vi "playback.vi"() -> ()   [LabVIEW 2012]
doc: "This VI will initialize the FPGA VI and read a user-defined number of samples from a DMA FIFO. When the data acquisition is complete this VI will read status information from the FPGA VI.\n\nFollow these instructions to run the VI.\n\n1. Select your RIO device from the dropdown.\n2. Set the sample period, number of samples to acquire per channel, and DMA block read size. \n\nNote: the block read size should be set to balance load on the host processor and the update rate of the user interface. A small block read size will update the user interface more often but will result in a higher load on the host processor."
uses:
  <vilib>/Analysis/3filter.llb/Butterworth Filter (DBL).vi
  <vilib>/Analysis/NI_AALBase.lvlib
  <vilib>/Analysis/NI_AALPro.lvlib
panel:
  in  "Wait?":bool
  in  "Filename":path=path "D:/Recorded/US Test/Record 1/Robosub.tdms"
  in  "Next Signal":bool
  in  "threshold ratio":dbl=3.0
  out "Sidemove":dbl
  out "Forward":dbl
  out "Threshold 3":dbl
  out "Threshold 2":dbl
  out "Threshold 1":dbl
  out "noise index":dbl[](array[numeric])
  out "Threshold 0":dbl
  out "Amplitude Spectrum":waveform(dbl)(graph)
  out "bad signal?":bool
  in  "Min Starting Index":i32=7000
  in  "Portion Duration":i32=1000
  out "amplitude 3":dbl
  out "amplitude 2":dbl
  out "amplitude 1":dbl
  out "amplitude 0":dbl
  in  "noise min":dbl=0.001
  out "Index 3":dbl
  out "Index 2":dbl
  out "Index 1":dbl
  out "Index 0":dbl
  in  "Send to ROS":bool
  out "ROS  Error":bool
  out "dt1":dbl
  out "dt2":dbl
  out "dt3":dbl
  out "pitch":dbl
  out "yaw":dbl
  out "z":dbl
  out "y":dbl format="%#_6f"
  out "x":dbl format="%#_6f"
  in  "Mode":T1(ring)=enum."Use Far Field"
  in  "Altitude":dbl=2.0
  in  "Display Filtered Signal":bool=TRUE
  out "Ratio at Index (%)":dbl
  out "Selected Index":i32
  in  "Threshold":dbl=0.1
  in  "low cutoff freq: fl":dbl=20000.0
  in  "high cutoff freq: fh":dbl=30000.0
  out "Yaw Chart":dbl(graph)
  out "Ch0 Signal":dbl[](graph)
  out "Extracted signal":dbl[][](graph)
  # "Peak Finding"
  # "Setpoints"
  # "TDOA (us)"
  # "Triangulation Result"
  # "Signal Processing Control"
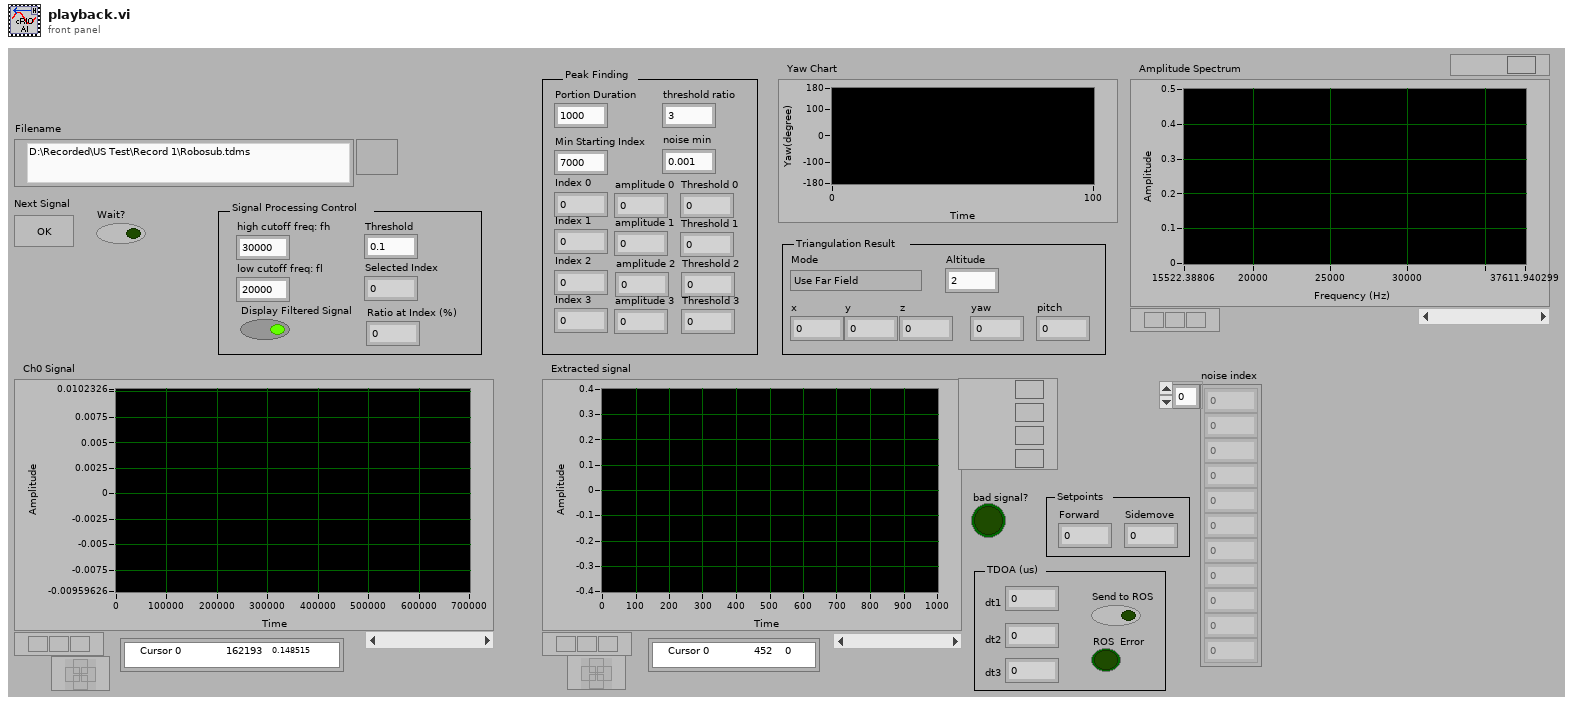
[diagram p1: front panel]
types:
  T1 = enum16{"Use Near Field", "Use Far Field", "Far Field with 3 hydrophones"}
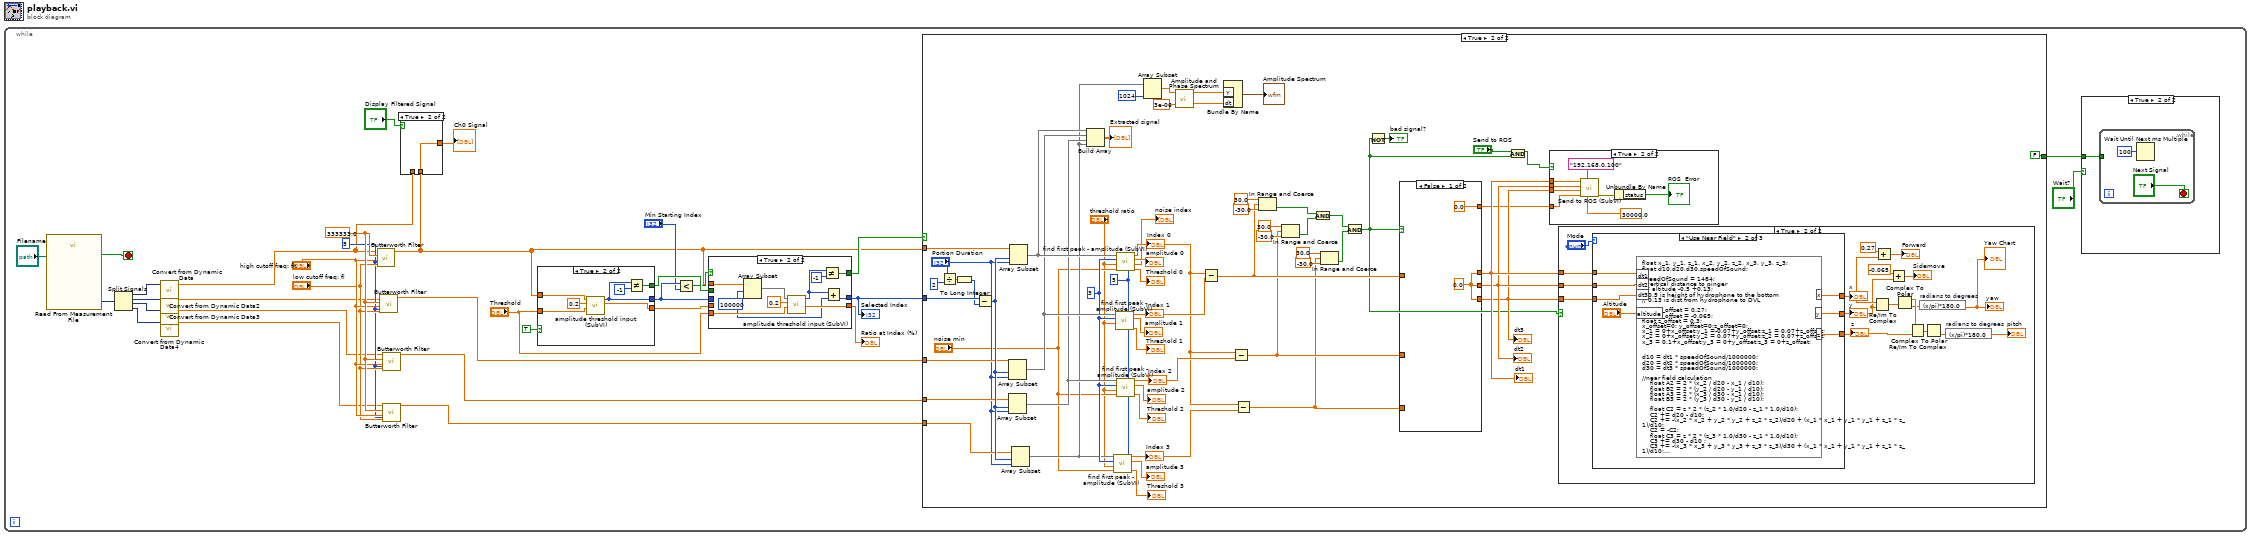
[diagram p0: block diagram]
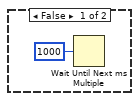
[diagram p2: hidden frame]
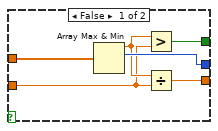
[diagram p5: hidden frame]
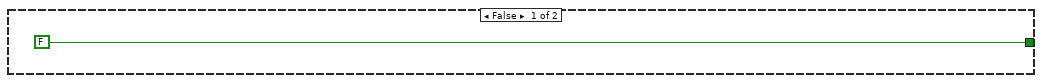
[diagram p6: hidden frame]
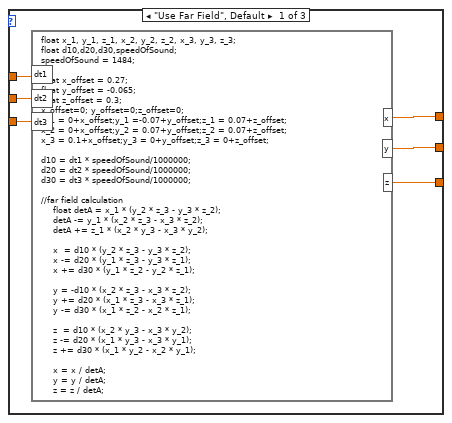
[diagram p8: hidden frame]
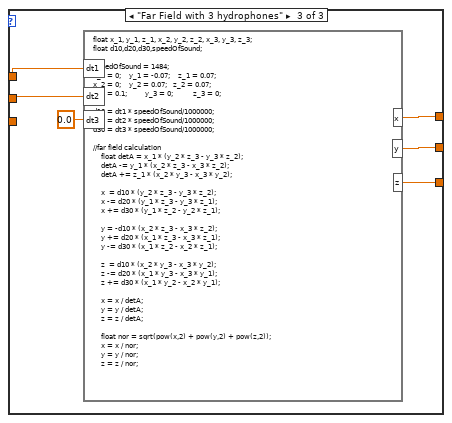
[diagram p9: hidden frame]
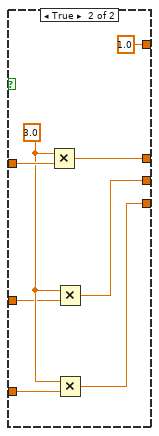
[diagram p11: hidden frame]
diagram:
  n1 = while {
    stop <- w6 stop-if-true
    w18 = 5 ("order")
    w24 = 333333.0 ("sampling freq: fs")
    n2 = call "Read From Measurement File"("Filename"="Filename") -> ("Signals"=w11:dynamicdata, "EOF?"=w6:bool)  [unwired: 5 in, 4 out]
    n3 = Split Signals(w11) -> (w15:dynamicdata, w14:dynamicdata, w13:dynamicdata, w12:dynamicdata)  [unwired: 4 in]
    n4 = call "Convert from Dynamic Data"("Dynamic Data Type"=w15) -> ("Array"=w10:dbl[])  [unwired: 3 in]
    n5 = call "Convert from Dynamic Data2"("Dynamic Data Type"=w14) -> ("Array"=w9:dbl[])  [unwired: 3 in]
    n6 = call "Convert from Dynamic Data3"("Dynamic Data Type"=w13) -> ("Array"=w7:dbl[])  [unwired: 3 in]
    n7 = call "Convert from Dynamic Data4"("Dynamic Data Type"=w12) -> ("Array"=w8:dbl[])  [unwired: 3 in]
    n8 = call-poly <vilib>:"Butterworth Filter.vi"("order"=w18, "low cutoff freq: fl"="low cutoff freq: fl", "high cutoff freq: fh"="high cutoff freq: fh", "sampling freq: fs"=w24, "X"=w10) -> ("Filtered X"=w16:dbl[])  [unwired: 3 in, 1 out]
    n9 = call-poly <vilib>:"Butterworth Filter.vi"("order"=w18, "low cutoff freq: fl"="low cutoff freq: fl", "high cutoff freq: fh"="high cutoff freq: fh", "sampling freq: fs"=w24, "X"=w9) -> ("Filtered X"=w21:dbl[])  [unwired: 3 in, 1 out]
    n10 = call-poly <vilib>:"Butterworth Filter.vi"("order"=w18, "low cutoff freq: fl"="low cutoff freq: fl", "high cutoff freq: fh"="high cutoff freq: fh", "sampling freq: fs"=w24, "X"=w8) -> ("Filtered X"=w19:dbl[])  [unwired: 3 in, 1 out]
    n11 = call-poly <vilib>:"Butterworth Filter.vi"("order"=w18, "low cutoff freq: fl"="low cutoff freq: fl", "high cutoff freq: fh"="high cutoff freq: fh", "sampling freq: fs"=w24, "X"=w7) -> ("Filtered X"=w20:dbl[])  [unwired: 3 in, 1 out]
    n12 = case shown="True" "Display Filtered Signal" {
      tunnel: w10 -> [w38 _]
      tunnel: [w38 w39] -> w4
      tunnel: w16 -> [_ w39]
      frame False {
      }
      frame True {
      }
    }
    "Ch0 Signal" <- w4
    n13 = case shown="True" TRUE {
      tunnel: w16 -> [w58 w65]
      tunnel: [w55 w62] -> w30
      tunnel: [w56 w61] -> w27
      tunnel: [w57 w60] -> w32
      tunnel: "Threshold" -> [w53 w59]
      frame False {
        n14 = Array Max & Min(array=w58) -> (max value=w54:dbl, max index (indices)=w56:i32)  [unwired: 2 out]
        n15 = Greater?(x=w54, y=w53) -> (0:w57:bool)
        n16 = Divide(x=w54, y=w53) -> (x/y=w55:dbl)
      }
      frame True {
        n17 = call "amplitude threshold input (SubVI).vi"("threshold"=w59, "%max amplitude"=0.2, "Array"=w65) -> ("actual ratio (%)"=w62:dbl, "Index"=w61:i32)  [unwired: 7 in]
        n18 = Not Equal?(x=w61, y=-1) -> (x != y?=w60:bool)
      }
    }
    n19 = Less?(x=w27, y="Min Starting Index") -> (x < y?=w31:bool)
    n20 = case shown="True" w31 {
      tunnel: w32 -> [w42 _]
      tunnel: w30 -> [w40 _]
      tunnel: w16 -> [_ w52]
      tunnel: "Threshold" -> [_ w48]
      tunnel: [w42 w47] -> w25
      tunnel: [w41 w45] -> w26
      tunnel: [w40 w46] -> w28
      tunnel: w27 -> [w41 _]
      frame False {
      }
      frame True {
        w43 = 100000 ("index")
        n21 = Array Subset(array=w52, index=w43) -> (w49:dbl[])  [unwired: 1 in]
        n22 = call "amplitude threshold input (SubVI).vi"("threshold"=w48, "%max amplitude"=0.2, "Array"=w49) -> ("actual ratio (%)"=w46:dbl, "Index"=w44:i32)  [unwired: 7 in]
        n23 = Not Equal?(x=w44, y=-1) -> (x != y?=w47:bool)
        n24 = Add(x=w44, y=w43) -> (x+y=w45:i32)
      }
    }
    "Ratio at Index (%)" <- w28
    "Selected Index" <- w26
    n25 = case shown="True" w25 {
      tunnel: w21 -> [_ w125]
      tunnel: w20 -> [_ w124]
      tunnel: w19 -> [_ w123]
      tunnel: w16 -> [_ w122]
      tunnel: w26 -> [_ w121]
      tunnel: [FALSE ("Debug") FALSE ("Debug")] -> w3
      frame False {
      }
      frame True {
        w74 = 5 ("Noise length")
        w87 = 3
        n26 = Divide(x="Portion Duration", y=2) -> (x/y=w118:dbl)
        n27 = To Long Integer(number=w118) -> (32bit integer=w117:i32)
        n28 = Subtract(x=w121, y=w117) -> (x-y=w126:i32)
        n29 = Array Subset(array=w124, index=w126, length="Portion Duration") -> (w88:dbl[])
        n30 = Array Subset(array=w125, index=w126, length="Portion Duration") -> (w92:dbl[])
        n31 = Array Subset(array=w122, index=w126, length="Portion Duration") -> (w94:dbl[])
        n32 = Array Subset(array=w123, index=w126, length="Portion Duration") -> (w86:dbl[])
        n33 = Build Array(w94, w92, w88, w86) -> (→"Extracted signal":dbl[][])
        n34 = call "find first peak - amplitude (SubVI).vi"("Noise length"=w74, "Noise min"="noise min", "threshold ratio"="threshold ratio", "width"=w87, "Array"=w86) -> ("Peak threshold"=→"Threshold 3":dbl, "peak amplitude"=→"amplitude 3":dbl, "Index"=w85:dbl)  [unwired: 2 in, 2 out]
        "Index 3" <- w85
        n35 = call "find first peak - amplitude (SubVI).vi"("Noise length"=w74, "threshold ratio"="threshold ratio", "width"=w87, "Array"=w92) -> ("Peak threshold"=→"Threshold 1":dbl, "peak amplitude"=→"amplitude 1":dbl, "Index"=w91:dbl)  [unwired: 3 in, 2 out]
        "Index 1" <- w91
        n36 = call "find first peak - amplitude (SubVI).vi"("Noise length"=w74, "Noise min"="noise min", "threshold ratio"="threshold ratio", "width"=w87, "Array"=w94) -> ("Peak threshold"=→"Threshold 0":dbl, "noise index"=→"noise index":dbl[], "peak amplitude"=→"amplitude 0":dbl, "Index"=w81:dbl)  [unwired: 2 in, 1 out]
        "Index 0" <- w81
        n37 = call "find first peak - amplitude (SubVI).vi"("Noise length"=w74, "Noise min"="noise min", "threshold ratio"="threshold ratio", "width"=w87, "Array"=w88) -> ("Peak threshold"=→"Threshold 2":dbl, "peak amplitude"=→"amplitude 2":dbl, "Index"=w89:dbl)  [unwired: 2 in, 2 out]
        "Index 2" <- w89
        n38 = Array Subset(array=w86, length=1024) -> (w70:dbl[])  [unwired: 1 in]
        n39 = call <vilib>:"Amplitude and Phase Spectrum.vi"("dt"=3e-06, "Signal (V)"=w70) -> ("df"=w67:dbl, "Amp Spectrum Mag (Vrms)"=w68:dbl[])  [unwired: 1 in, 1 out]
        n40 = Subtract(x=w81, y=w91) -> (x-y=w113:dbl)
        n41 = Bundle By Name("Y"=w68, "dt"=w67) -> (→"Amplitude Spectrum":waveform(dbl))  [unwired: 1 in]
        n42 = Subtract(x=w81, y=w89) -> (x-y=w110:dbl)
        n43 = Subtract(x=w81, y=w85) -> (x-y=w107:dbl)
        n44 = In Range and Coerce(upper limit=30.0, x=w113, lower limit=-30.0) -> (In Range?=w106:bool)  [unwired: 1 out]
        n45 = In Range and Coerce(upper limit=30.0, x=w110, lower limit=-30.0) -> (In Range?=w105:bool)  [unwired: 1 out]
        n46 = And(x=w106, y=w105) -> (x .and. y?=w104:bool)
        n47 = In Range and Coerce(upper limit=30.0, x=w107, lower limit=-30.0) -> (In Range?=w103:bool)  [unwired: 1 out]
        n48 = And(x=w104, y=w103) -> (x .and. y?=w95:bool)
        n49 = Not(x=w95) -> (.not. x?=→"bad signal?":bool)
        n50 = case shown="False" w95 {
          tunnel: w113 -> [_ w181]
          tunnel: w110 -> [_ w179]
          tunnel: w107 -> [_ w178]
          tunnel: [w172 w177] -> w100
          tunnel: [w172 w176] -> w99
          tunnel: [w172 w175] -> w98
          tunnel: [0.0 ("x") 1.0 ("x")] -> w97
          frame False {
            w172 = 0.0
          }
          frame True {
            w180 = 3.0 ("x")
            n51 = Multiply(x=w180, y=w181) -> (x*y=w177:dbl)
            n52 = Multiply(x=w180, y=w179) -> (x*y=w176:dbl)
            n53 = Multiply(x=w180, y=w178) -> (x*y=w175:dbl)
          }
        }
        "dt1" <- w100
        "dt2" <- w99
        "dt3" <- w98
        n54 = And(x="Send to ROS", y=w95) -> (x .and. y?=w96:bool)
        n55 = case shown="True" w96 {
          tunnel: w100 -> [_ w167]
          tunnel: w99 -> [_ w166]
          tunnel: w98 -> [_ w165]
          tunnel: w97 -> [_ w164]
          frame False {
          }
          frame True {
            n56 = call "Send to ROS (SubVI).vi"("frequency"=30000.0, "ROS IP"="192.168.0.100", "Good signal?"=w164, "dt 3"=w165, "dt2"=w166, "dt 1"=w167) -> ("error out"=w170:errorcluster)  [unwired: 5 in]
            n57 = Unbundle By Name(w170) -> ("status"=→"ROS  Error":bool)
          }
        }
        n58 = case shown="True" w95 {
          tunnel: w100 -> [_ w135]
          tunnel: w99 -> [_ w134]
          tunnel: w98 -> [_ w133]
          frame False {
          }
          frame True {
            n59 = case shown="\"Use Near Field\"" "Mode" {
              tunnel: [w150 w157 w162] -> w132
              tunnel: [w149 w156 w161] -> w129
              tunnel: [w148 w155 w160] -> w139
              tunnel: w135 -> [w147 w153 w159]
              tunnel: w134 -> [w146 w152 w158]
              tunnel: w133 -> [w145 w151 _]
              frame "Use Far Field", Default {
                n60 = formula code="float x_1, y_1, z_1, x_2, y_2, z_2, x_3, y_3, z_3;\nfloat d10,d20,d30,speedOfSound;\nspeedOfSound = 1484;\n\nfloat x_offset = 0.27;\nfloat y_offset = -0.065;\nfloat z_offset = 0.3;\nx_offset=0; y_offset=0;z_offset=0;\nx_1 = 0+x_offset;y_1 =-0.07+y_offset;z_1 = 0.07+z_offset;\nx_2 = 0+x_offset;y_2 = 0.07+y_offset;z_2 = 0.07+z_offset;\nx_3 = 0.1+x_offset;y_3 = 0+y_offset;z_3 = 0+z_offset;\n\nd10 = dt1 * speedOfSound/1000000;\nd20 = dt2 * speedOfSound/1000000;\nd30 = dt3 * speedOfSound/1000000;\n\n//far field calculation\n    float detA = x_1 * (y_2 * z_3 - y_3 * z_2);\n    detA -= y_1 * (x_2 * z_3 - x_3 * z_2);\n    detA += z_1 * (x_2 * y_3 - x_3 * y_2);\n\n    x  = d10 * (y_2 * z_3 - y_3 * z_2);\n    x -= d20 * (y_1 * z_3 - y_3 * z_1);\n    x += d30 * (y_1 * z_2 - y_2 * z_1);\n\n    y = -d10 * (x_2 * z_3 - x_3 * z_2);\n    y += d20 * (x_1 * z_3 - x_3 * z_1);\n    y -= d30 * (x_1 * z_2 - x_2 * z_1);\n\n    z  = d10 * (x_2 * y_3 - x_3 * y_2);\n    z -= d20 * (x_1 * y_3 - x_3 * y_1);\n    z += d30 * (x_1 * y_2 - x_2 * y_1);\n\n    x = x / detA;\n    y = y / detA;\n    z = z / detA;\n\n    float nor = sqrt(pow(x,2) + pow(y,2) + pow(z,2));\n    x = x / nor;\n    y = y / nor;\n    z = z / nor;"("dt1"=w147, "dt2"=w146, "dt3"=w145) -> ("x"=w150:dbl, "y"=w149:dbl, "z"=w148:dbl)
              }
              frame "Use Near Field" {
                n61 = formula code="float x_1, y_1, z_1, x_2, y_2, z_2, x_3, y_3, z_3;\nfloat d10,d20,d30,speedOfSound;\n\nspeedOfSound = 1484;\n//vertical distance to pinger\nz= altitude -0.5 +0.13;\n// 0.5 is height of hydrophone to the bottom\n// 0.13 is dist from hydrophone to DVL\n\nfloat x_offset = 0.27;\nfloat y_offset = -0.065;\nfloat z_offset = 0.3;\nx_offset=0; y_offset=0;z_offset=0;\nx_1 = 0+x_offset;y_1 =-0.07+y_offset;z_1 = 0.07+z_offset;\nx_2 = 0+x_offset;y_2 = 0.07+y_offset;z_2 = 0.07+z_offset;\nx_3 = 0.1+x_offset;y_3 = 0+y_offset;z_3 = 0+z_offset;\n\n\nd10 = dt1 * speedOfSound/1000000;\nd20 = dt2 * speedOfSound/1000000;\nd30 = dt3 * speedOfSound/1000000;\n\n//near field calculation\n    float A2 = 2 * (x_2 / d20 - x_1 / d10);\n    float B2 = 2 * (y_2 / d20 - y_1 / d10);\n    float A3 = 2 * (x_3 / d30 - x_1 / d10);\n    float B3 = 2 * (y_3 / d30 - y_1 / d10);\n    \n    float C2 = z * 2 * (z_2 * 1.0/d20 - z_1 * 1.0/d10);\n    C2 += d20 - d10;\n    C2 += -(x_2 * x_2 + y_2 * y_2 + z_2 * z_2)/d20 + (x_1 * x_1 + y_1 * y_1 + z_1 * z_1)/d10;\n    C2 = -C2;\n    float C3 = z * 2 * (z_3 * 1.0/d30 - z_1 * 1.0/d10);\n    C3 += d30 - d10 ;\n    C3 += -(x_3 * x_3 + y_3 * y_3 + z_3 * z_3)/d30 + (x_1 * x_1 + y_1 * y_1 + z_1 * z_1)/d10;\n    C3 = -C3;\n\n    if (A2*B3 == A3*B2) {\n        x = 0;\n        y = 0;\n    }\n    else {\n        x = (C2 * B3 - C3 * B2) / (A2 * B3 - A3 * B2);\n        y = (C3 * A2 - C2 * A3) / (B3 * A2 - B2 * A3);\n    }"("dt1"=w153, "dt2"=w152, "dt3"=w151, "altitude"="Altitude") -> ("x"=w157:dbl, "y"=w156:dbl, "z"=w155:dbl)
              }
              frame "Far Field with 3 hydrophones" {
                n62 = formula code="float x_1, y_1, z_1, x_2, y_2, z_2, x_3, y_3, z_3;\nfloat d10,d20,d30,speedOfSound;\n\nspeedOfSound = 1484;\nx_1 = 0;    y_1 = -0.07;    z_1 = 0.07;\nx_2 = 0;    y_2 = 0.07;   z_2 = 0.07;\nx_3 = 0.1;         y_3 = 0;          z_3 = 0;\n\nd10 = dt1 * speedOfSound/1000000;\nd20 = dt2 * speedOfSound/1000000;\nd30 = dt3 * speedOfSound/1000000;\n\n//far field calculation\n    float detA = x_1 * (y_2 * z_3 - y_3 * z_2);\n    detA -= y_1 * (x_2 * z_3 - x_3 * z_2);\n    detA += z_1 * (x_2 * y_3 - x_3 * y_2);\n\n    x  = d10 * (y_2 * z_3 - y_3 * z_2);\n    x -= d20 * (y_1 * z_3 - y_3 * z_1);\n    x += d30 * (y_1 * z_2 - y_2 * z_1);\n\n    y = -d10 * (x_2 * z_3 - x_3 * z_2);\n    y += d20 * (x_1 * z_3 - x_3 * z_1);\n    y -= d30 * (x_1 * z_2 - x_2 * z_1);\n\n    z  = d10 * (x_2 * y_3 - x_3 * y_2);\n    z -= d20 * (x_1 * y_3 - x_3 * y_1);\n    z += d30 * (x_1 * y_2 - x_2 * y_1);\n\n    x = x / detA;\n    y = y / detA;\n    z = z / detA;\n\n    float nor = sqrt(pow(x,2) + pow(y,2) + pow(z,2));\n    x = x / nor;\n    y = y / nor;\n    z = z / nor;"("dt1"=w159, "dt2"=w158, "dt3"=0.0 ("input variable")) -> ("x"=w162:dbl, "y"=w161:dbl, "z"=w160:dbl)
              }
            }
            "x" <- w132
            "y" <- w129
            "z" <- w139
            n63 = Re/Im To Complex(1:w129, 2:w132) -> (0:w137:cdb)
            n64 = Add(x=0.27, y=w132) -> (x+y=→"Forward":dbl)
            n65 = Add(x=-0.065, y=w129) -> (x+y=→"Sidemove":dbl)
            n66 = Complex To Polar(r * e^(i*theta)=w137) -> (r=w140:dbl, theta=w138:dbl)
            n67 = Re/Im To Complex(1:w139, 2:w140) -> (0:w141:cdb)
            n68 = expression code="(x/pi)*180.0" "radians to degrees"(w138) -> (→"yaw" →"Yaw Chart":dbl)
            n69 = Complex To Polar(r * e^(i*theta)=w141) -> (theta=w143:dbl)  [unwired: 1 out]
            n70 = expression code="(x/pi)*180.0" "radians to degrees"(w143) -> (→"pitch":dbl)
          }
        }
      }
    }
    n71 = case shown="True" "Wait?" {
      tunnel: w3 -> [_ w35]
      frame False {
        n72 = Wait Until Next ms Multiple(millisecond multiple=u32 1000) -> ()  [unwired: 1 out]
      }
      frame True {
        n73 = while {
          tunnel: w35 -> [_]
          stop <- "Next Signal" stop-if-true
          n74 = Wait Until Next ms Multiple(millisecond multiple=u32 100) -> ()  [unwired: 1 out]
        }
      }
    }
  }
